vi "getAlignement.vi"(8 "error in (no error)":errorcluster, 11 "xwpfRun.Title in":refnum<class "xwpfRun.Title.lvclass">) -> (0 "error out":errorcluster, 2 "Alignment":u16(ring)=2 items=["LEFT"=1, "CENTER"=2, "RIGHT"=3, "BOTH"=4, "MEDIUM_KASHIDA"=5, "DISTRIBUTE"=6, "NUM_TAB"=7, "HIGH_KASHIDA"=8, "LOW_KASHIDA"=9, "THAI_DISTRIBUTE"=10], 3 "xwpfRun.Title out":refnum<class "xwpfRun.Title.lvclass">)   [LabVIEW 2017, in "Word_Specific.lvlib" / "xwpfRun.Title.lvclass"]
uses:
  xwpfRun.Title.lvclass
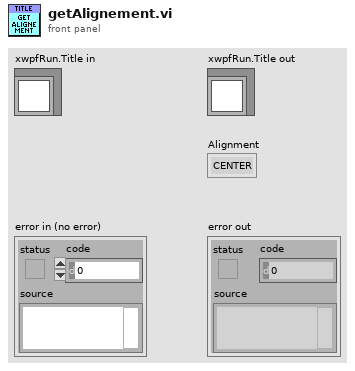
[diagram p1: front panel]
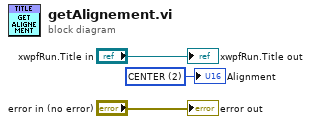
[diagram p0: block diagram]
diagram:
  w1 = u16 2 items=["LEFT"=1, "CENTER"=2, "RIGHT"=3, "BOTH"=4, "MEDIUM_KASHIDA"=5, "DISTRIBUTE"=6, "NUM_TAB"=7, "HIGH_KASHIDA"=8, "LOW_KASHIDA"=9, "THAI_DISTRIBUTE"=10] ("Alignment")
  "error out" <- "error in (no error)"
  "xwpfRun.Title out" <- "xwpfRun.Title in"
  "Alignment" <- w1
